vi "Advanced Custom Sensor Regulation.vi"() -> ()   [LabVIEW 2016]
doc: "This example shows how to use a custom sensor, different from Fluigent ones and regulate pressure in order to reach setpoint. Different sensor type and range can be used (e.g. liquid pressure, water level, l/min flow meter...) however we do not guarantee full compatibility with all sensors.\n\nFor this demonstration a Fluigent flow-unit is used for more simplicity.\n\nHardware setup: At least one Fluigent pressure controller (MFCS, MFCS-EZ or FlowEZ) and at least one Fluigent sensor (flow-unit connected to FRP or FlowEZ)"
uses:
  fgt_SDK.lvlib
panel:
  in  "Stop":bool
  out "Flowrate":cluster{"element":sgl, "pressure out":sgl}(graph)
  out "error out":errorcluster
  # "Hit the \"run\" button to start the regulation"
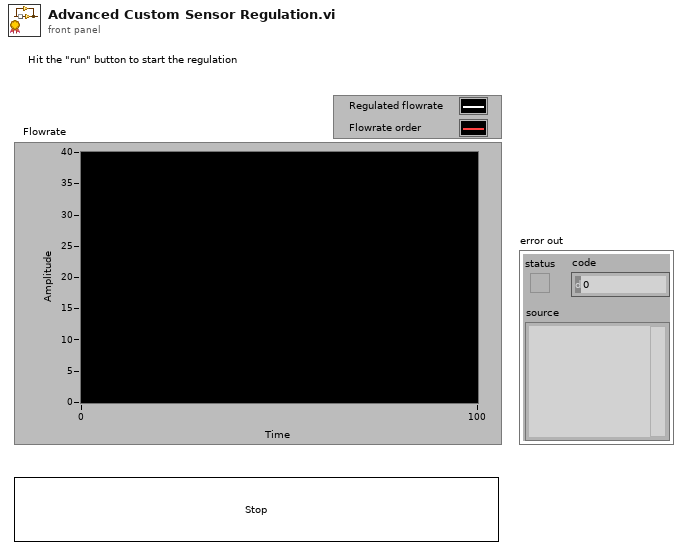
[diagram p1: front panel]
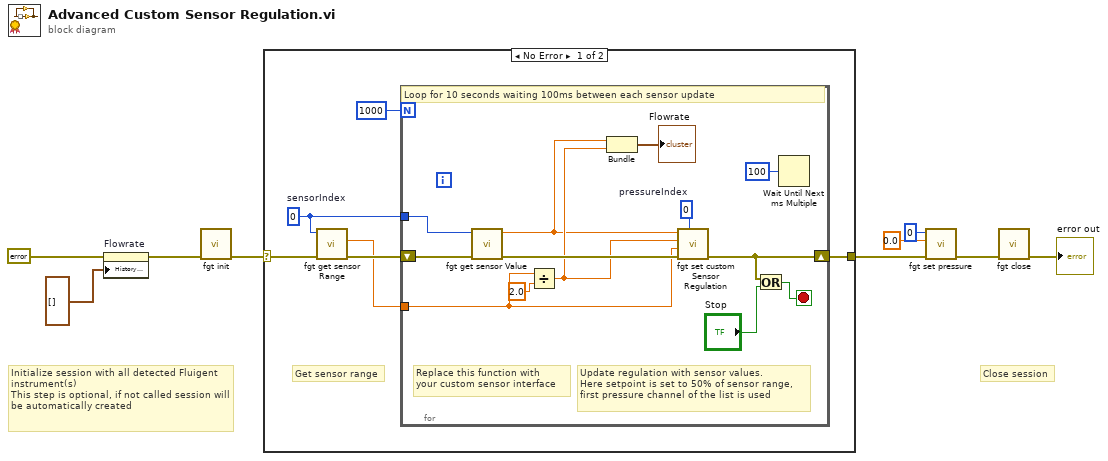
[diagram p0: block diagram]
diagram:
  # "Close session"
  # "Initialize session with all detected Fluigent instrument(s)\nThis step is optional, if not called session will be automatically created"
  n1 = property on="Flowrate" class="WFChart (strict)"(error in=errorcluster {"status"=FALSE, "code"=0, "source"=""} ("error in (no error)"), "History Data"=cluster{"element":sgl, "pressure out":sgl}[] []) -> (error out=w7:errorcluster)  [unwired: 1 in, 1 out]
  n2 = call "fgt init.vi"("error in (no error)"=w7) -> ("error out"=w9:errorcluster)  [unwired: 10 in]
  n3 = case shown="No Error" w9 {
    selector: w9 -> [w15 w29]
    tunnel: [w10 w29] -> w2
    frame No Error {
      w12 = u32 0  # sensorIndex
      # "Get sensor range"
      n4 = call "fgt get sensor Range.vi"("error in (no error)"=w15, "sensorIndex"=w12) -> ("error out"=w13:errorcluster, "Smax out"=w11:sgl)  [unwired: 7 in, 1 out]
      n5 = for {
        N: 1000 -> [_]
        shift-right: [w17] -> w10
        shift-left: w13 -> [w27]
        tunnel: w12 -> [w26]
        tunnel: w11 -> [w23]
        stop <- w18 stop-if-true
        w25 = u32 0  # pressureIndex
        # "Update regulation with sensor values. \nHere setpoint is set to 50% of sensor range, \nfirst pressure channel of the list is used"
        # "Replace this function with \nyour custom sensor interface"
        # "Loop for 10 seconds waiting 100ms between each sensor update"
        n6 = call "fgt get sensor Value.vi"("error in (no error)"=w27, "sensorIndex"=w26) -> ("error out"=w24:errorcluster, "value out"=w20:sgl)  [unwired: 8 in]
        n7 = Divide(x=w23, y=sgl 2.0) -> (x/y=w21:sgl)
        n8 = Bundle("value out"=w20, w21) -> (→"Flowrate":cluster{"value out":sgl, sgl})  [unwired: 1 in]
        n9 = call "fgt set custom Sensor Regulation.vi"("pressureIndex"=w25, "error in (no error)"=w24, "maxSensorRange"=w23, "setpoint"=w21, "measure"=w20) -> ("error out"=w17:errorcluster)  [unwired: 6 in]
        n10 = Or(x=w17, y="Stop") -> (x .or. y?=w18:bool)
        n11 = Wait Until Next ms Multiple(millisecond multiple=u32 100) -> ()  [unwired: 1 out]
      }
    }
    frame Error {
    }
  }
  n12 = call "fgt set pressure.vi"("error in (no error)"=w2, "pressure"=sgl 0.0, "pressureIndex"=u32 0) -> ("error out"=w1:errorcluster)  [unwired: 8 in]
  n13 = call "fgt close.vi"("error in (no error)"=w1) -> ("error out"=→"error out":errorcluster)  [unwired: 10 in]
